vi "Check and Override Channel Configuration.vi"(8 "error in (no error)":errorcluster, 10 "Custom Config Data in":u8[](array[numeric]) format="%.0x", 11 "CIF_Fifo_CAN in":refnum<class "CIF_CIPC_CAN.lvclass">) -> (0 "error out":errorcluster, 2 "Custom Config Data out":u8[](array[numeric]) format="%.0x", 3 "CIF_Fifo_CAN out":refnum<class "CIF_CIPC_CAN.lvclass">)   [LabVIEW 2021, in "CIF_CIPC_CAN.lvclass"]
uses:
  CIF_CIPC_CAN.lvclass
  <vilib>/CIF Foundation/CIF Utilities/DataTypes/Flatten Unflatten/Unflatten U64.vi
  <vilib>/CIF Foundation/CIF Utilities/DataTypes/Flatten Unflatten/Flatten U64.vi
  CIF_CIPC_CAN.lvclass/CIF_CIPC_CAN.ctl
  ChannelCommon/ChannelCommon.lvlib
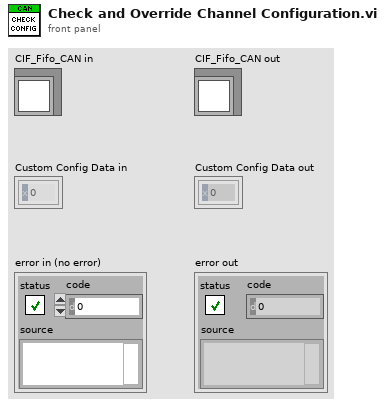
[diagram p1: front panel]
types:
  T1 = typedef "ChannelCommon.lvlib/FIFO Config.ctl" = cluster{"Max Bytes/Msg":u64, "Max Msg/FIFO":u64, "Flags":u64}
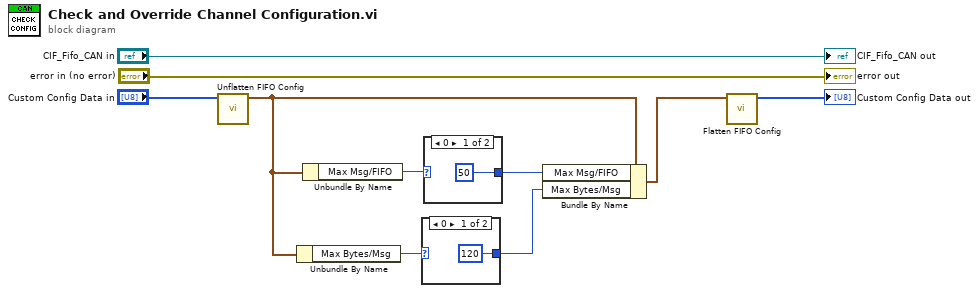
[diagram p0: block diagram]
diagram:
  n1 = call "Unflatten FIFO Config.vi"("Flattened Data in"="Custom Config Data in") -> ("FIFO Config out"=w4:T1)  [unwired: 9 in, 1 out]
  n2 = Unbundle By Name(w4) -> ("Max Bytes/Msg"=w6:u64)
  n3 = Unbundle By Name(w4) -> ("Max Msg/FIFO"=w5:u64)
  n4 = case shown="0" w6 {
    selector: w6 -> [_ w12]
    tunnel: [u64 120 ("y") w12] -> w1
    frame 0 {
    }
    frame 1, Default {
    }
  }
  n5 = case shown="0" w5 {
    selector: w5 -> [_ w14]
    tunnel: [u64 50 ("y") w14] -> w2
    frame 0 {
    }
    frame 1, Default {
    }
  }
  n6 = Bundle By Name(cluster=w4, "Max Msg/FIFO"=w2, "Max Bytes/Msg"=w1) -> (w3:T1)
  n7 = call "Flatten FIFO Config.vi"("FIFO Config in"=w3) -> ("Flattened FIFO Config"=→"Custom Config Data out":u8[])  [unwired: 10 in]
  "error out" <- "error in (no error)"
  "CIF_Fifo_CAN out" <- "CIF_Fifo_CAN in"
